vi "Chamber Engine.vi"(11 "Sequence Context In":refnum<k7>) -> (0 "error out":errorcluster)   [LabVIEW 2023, in "LTT_TeststandSteptypes.lvlib"]
uses:
  LTT_TeststandSteptypes.lvlib
  HardwareAbstractionLayer_LVOOP/Modbus TCP/Modbus TCP_class/Modbus TCP.lvclass
  Temperature Controller/Control/TC FGV Action.ctl
  75a4899f-3d6f-49ef-a0cc-877733f6873c.vi
  <vilib>/addons/TestStand/_TSUtility.llb/TestStand - Get Property Value (Boolean).vi
  GlobalVariable/GlobalVariableData.vi
  <vilib>/addons/TestStand/_TSUtility.llb/TestStand - Set Property Value (Number).vi
  HardwareAbstractionLayer_LVOOP/Teststand/Teststand.lvclass
  HardwareAbstractionLayer_LVOOP/Database/Database.lvclass
  HardwareAbstractionLayer_LVOOP/Modbus/Modbus_class/Modbus.lvclass
  HardwareAbstractionLayer_LVOOP/Database/SQL Public VI/Control/DB Options.ctl
panel:
  in  "stop":bool
  in  "error in (no error)":errorcluster
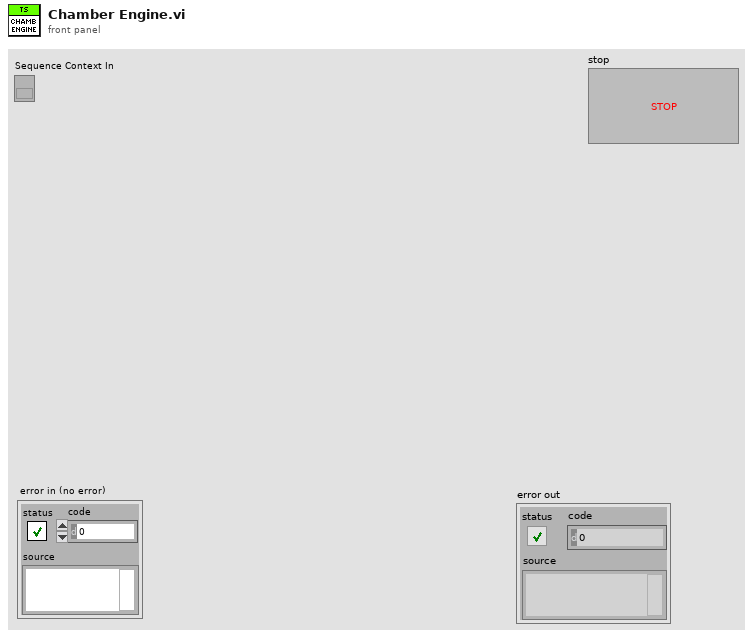
[diagram p1: front panel]
types:
  T1 = typedef "HardwareAbstractionLayer_LVOOP.lvlib/Database.lvclass/DB Options.ctl" = enum16{"Init", "Select Data", "Insert Data", "Update Data", "Delete Data", "Execute Query", "Create Schema", "Create Table", "List Tables", "List Columns", "Close"}
  T2 = typedef "LTT_TeststandSteptypes.lvlib/TC FGV Action.ctl" = enum16{"Set", "Get"}
  T3 = typedef "TestStand - Status Monitor.ctl" = cluster{"Sequence Context":refnum<k7>, "Execution":refnum<k7>, "Termination Monitor":refnum<k7>}
  T4 = typedef "HardwareAbstractionLayer_LVOOP.lvlib/Report.lvclass/Temperature LOG.ctl" = cluster{"TEST_MODE":string, "CYCLE_NUMBER":string, "TEMPERATURE":cluster{"LV_PPS_TEMPERATURE":dbl, "HV_PPS1_TEMPERATURE":dbl, "HV_PPS2_TEMPERATURE":dbl, "HV_PPS3_TEMPERATURE":dbl, "HV_PPS4_TEMPERATURE":dbl, "HV_PPS5_TEMPERATURE":dbl, "HV_PPS6_TEMPERATURE":dbl, "CHAMBER_TEMPERATURE":dbl, "LOAD_U1_TEMPERATURE":dbl, "LOAD_V1_TEMPERATURE":dbl, "LOAD_W1_TEMPERATURE":dbl, "LOAD_U2_TEMPERATURE":dbl, "LOAD_V2_TEMPERATURE":dbl, "LOAD_W2_TEMPERATURE":dbl, "LOAD_U3_TEMPERATURE":dbl, "LOAD_V3_TEMPERATURE":dbl, "LOAD_W3_TEMPERATURE":dbl}, "Temperature Inrange":cluster{"LVPPS_Trip?":bool, "HVPPS1_Trip?":bool, "HVPPS2_Trip?":bool, "HVPPS3_Trip?":bool, "HVPPS4_Trip?":bool, "HVPPS5_Trip?":bool, "HVPPS6_Trip?":bool, "Chamber_Trip?":bool}}
  T5 = cluster{"Chamber Present Temp":dbl, "Chamber Target Temp":dbl, "Chamber RTD Temp":dbl}
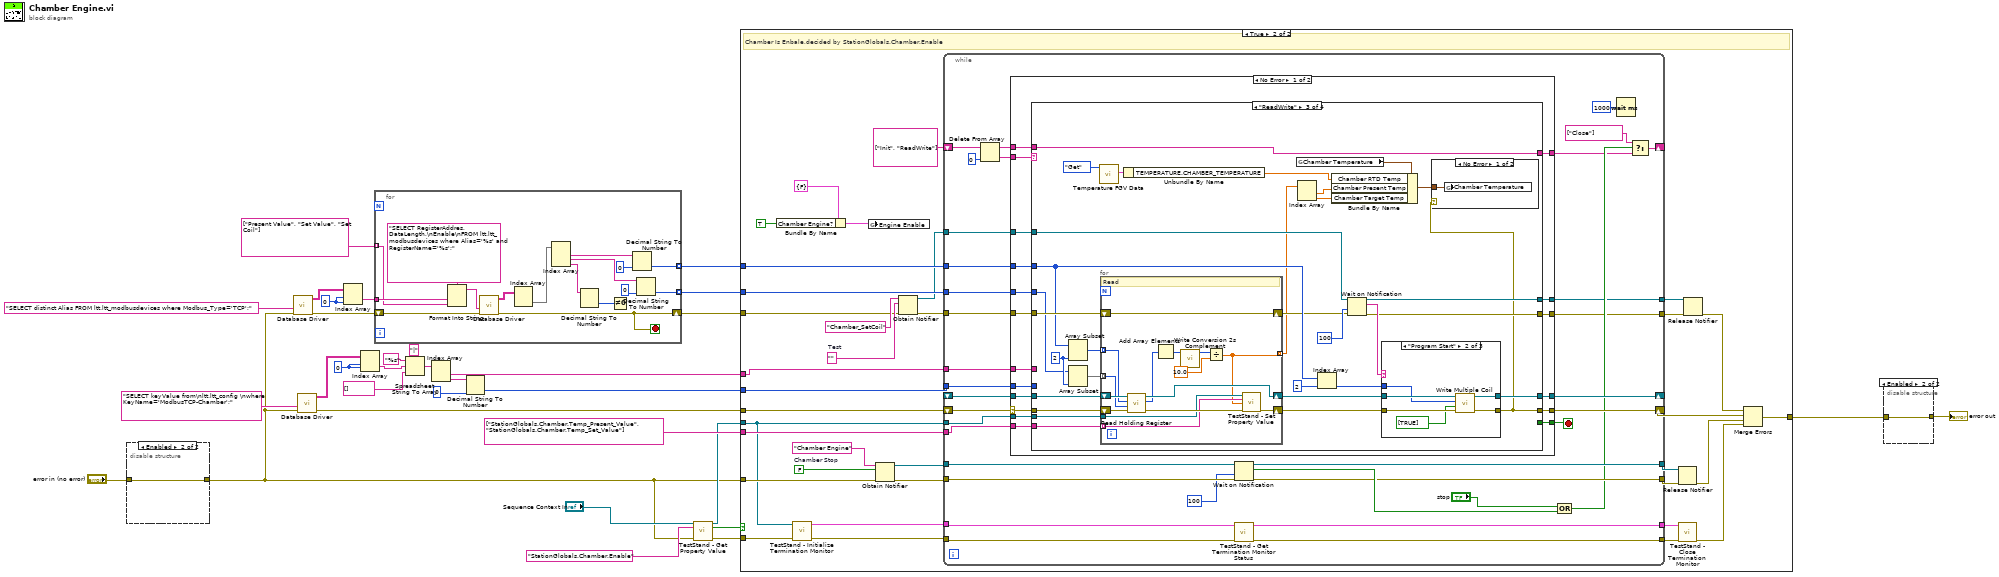
[diagram p0: block diagram]
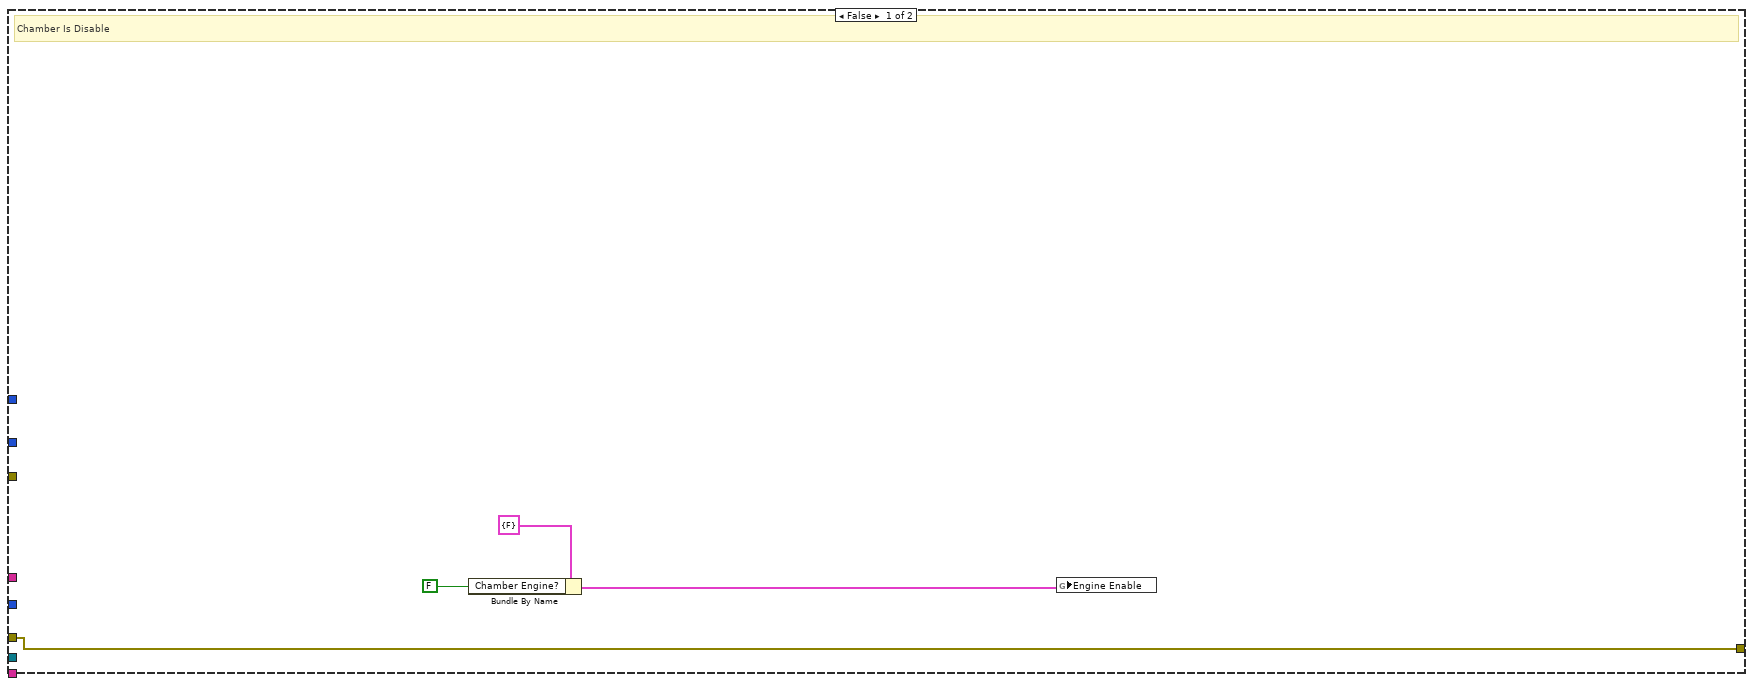
[diagram p2: hidden frame]
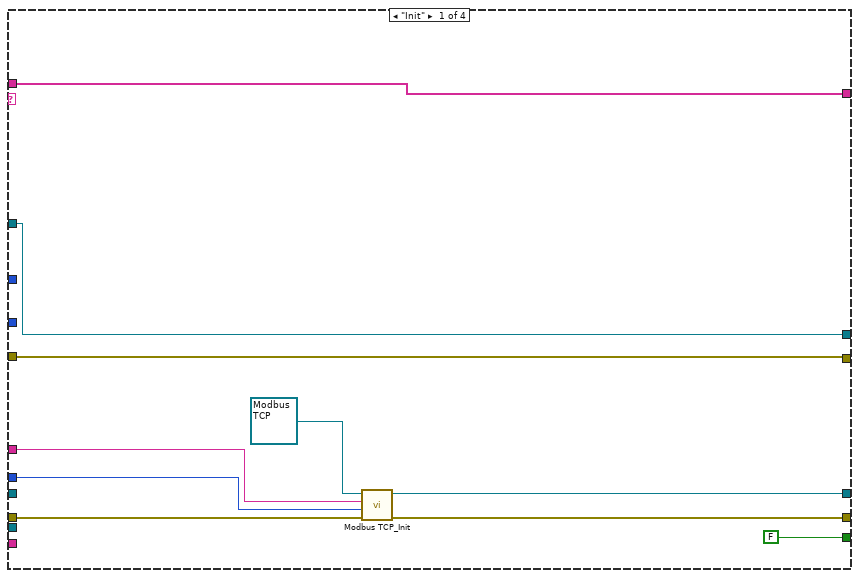
[diagram p3: hidden frame]
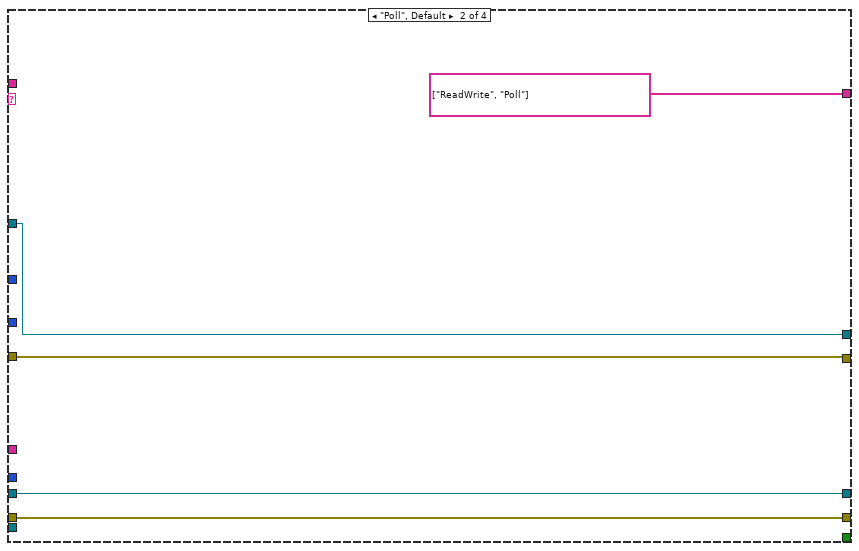
[diagram p4: hidden frame]
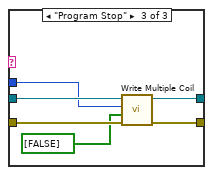
[diagram p7: hidden frame]
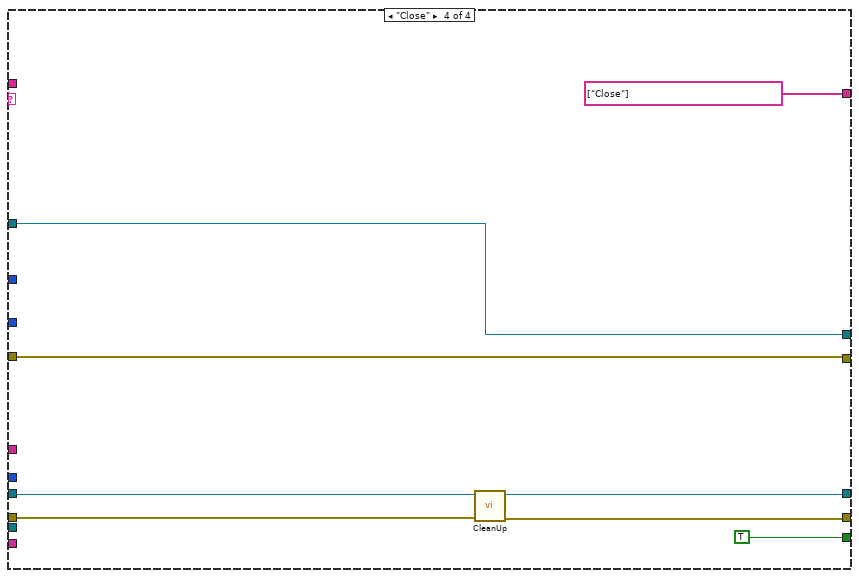
[diagram p8: hidden frame]
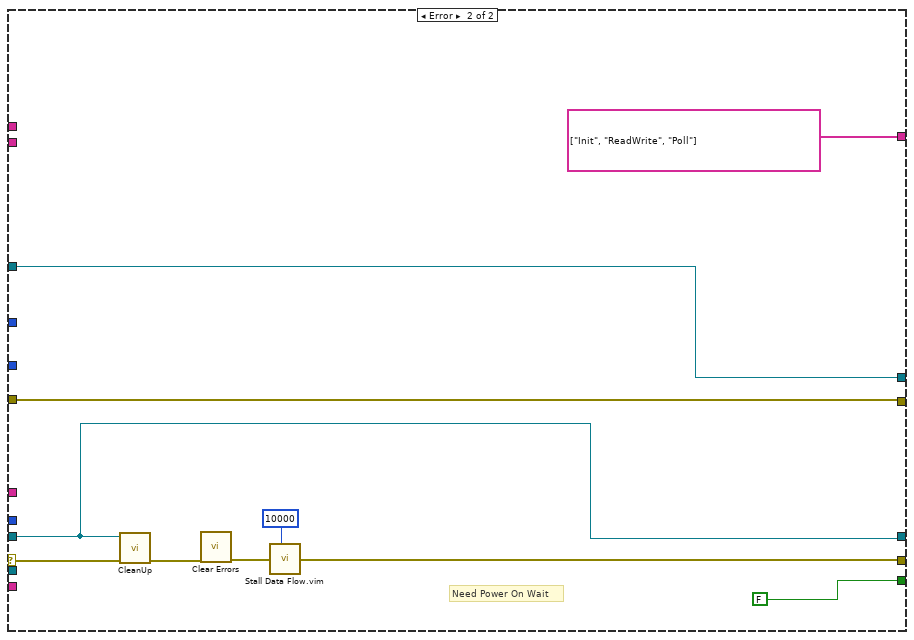
[diagram p9: hidden frame]
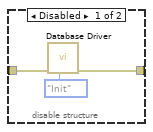
[diagram p10: hidden frame]
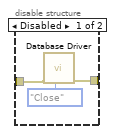
[diagram p11: hidden frame]
diagram:
  w17 = 0 ("disabled index (col)")
  w25 = 0 ("index (row)")
  n1 = disable-structure shown="Enabled" {
    disable-tunnel: "error in (no error)" -> [w34 w36]
    disable-tunnel: [w33 w36] -> w3
    frame Disabled {
      n2 = call "Database Driver.vi"("Options"=DB_Options."Init", "error in"=w34) -> ("error out"=w33:errorcluster)  [unwired: 6 in, 3 out]
    }
    frame Enabled {
    }
  }
  n3 = call "Database Driver.vi"("error in"=w3, "SQL query"="SELECT distinct Alias FROM ltt.ltt_modbusdevices where Modbus_Type='TCP';") -> ("error out"=w16:errorcluster, "data"=w18:string[][])  [unwired: 6 in, 2 out]
  n4 = call "Database Driver.vi"("error in"=w3, "SQL query"="SELECT keyValue from\nltt.ltt_config \nwhere KeyName='ModbusTCP-Chamber';") -> ("error out"=w20:errorcluster, "data"=w26:string[][])  [unwired: 6 in, 2 out]
  n5 = Index Array(array=w18, index (row)=w17, index (col)=w17) -> (element=w19:string)
  n6 = Index Array(array=w26, index (row)=w25, index (col)=w25) -> (element=w32:string)
  n7 = for {
    tunnel: w19 -> [w40]
    tunnel: [w46] -> w14 mode=indexing
    tunnel: [w45] -> w13 mode=indexing
    shift-right: [w44] -> w12
    shift-left: w16 -> [w43]
    tunnel: string[] ["Present Value", "Set Value", "Set Coil"] -> [w39] mode=indexing
    stop <- w44 stop-if-true
    n8 = Format Into String(format string="SELECT RegisterAddres, DataLength,\nEnable\nFROM ltt.ltt_modbusdevices where Alias='%s' and RegisterName='%s';", w40, w39) -> (resulting string=w52:string)  [unwired: 2 in, 1 out]
    n9 = call "Database Driver.vi"("error in"=w43, "SQL query"=w52) -> ("error out"=w44:errorcluster, "data"=w51:string[][])  [unwired: 6 in, 2 out]
    n10 = Index Array(array=w51) -> (element=w50:string[])  [unwired: 2 in]
    n11 = Index Array(array=w50) -> (element #1=w42:string, element #2=w41:string, element #3=w38:string)  [unwired: 3 in]
    n12 = Decimal String To Number(string=w38) -> (number=w37:i32)  [unwired: 2 in, 1 out]
    n13 = Not Equal To 0?(x=w37) -> ()  [unwired: 1 out]
    n14 = Decimal String To Number(string=w42, default (0L)=u16 0 ("starting address")) -> (number=w46:u16)  [unwired: 1 in, 1 out]
    n15 = Decimal String To Number(string=w41, default (0L)=u16 0 ("number of inputs")) -> (number=w45:u16)  [unwired: 1 in, 1 out]
  }
  n16 = Spreadsheet String To Array(delimiter (Tab)="|" ("format string"), format string="%s", spreadsheet string=w32, array type (2D Dbl)=string[] []) -> (array=w30:string[])
  n17 = Index Array(array=w30) -> (element #1=w21:string, element #2=w23:string)  [unwired: 2 in]
  n18 = Decimal String To Number(string=w23, default (0L)=u16 0 ("Port")) -> (number=w22:u16)  [unwired: 1 in, 1 out]
  n19 = call-poly <vilib>:"TestStand - Get Property Value.vi"("Sequence Context In"="Sequence Context In", "Lookup String"="StationGlobals.Chamber.Enable", "error in (no error)"=w3) -> ("Sequence Context Out"=w5:refnum<k7>, "Value"=w1:bool, "error out"=w2:errorcluster)  [unwired: 10 in]
  n20 = case shown="True" w1 {
    tunnel: w22 -> [_ w77]
    tunnel: w21 -> [_ w76]
    tunnel: w20 -> [w55 w75]
    tunnel: w14 -> [_ w74]
    tunnel: w13 -> [_ w73]
    tunnel: w12 -> [_ w70]
    tunnel: w3 -> [_ w64]
    tunnel: [w55 w63] -> w9
    tunnel: string[] ["StationGlobals.Chamber.Temp_Present_Value", "StationGlobals.Chamber.Temp_Set_Value"] -> [_ w59]
    tunnel: w5 -> [_ w56]
    tunnel: w2 -> [_ w57]
    frame False {
      w54 = cluster{"Chamber Engine?":bool} {"Chamber Engine?"=FALSE} ("Engine Enable")
      # "Chamber Is Disable"
      n21 = Bundle By Name(cluster=w54, "Chamber Engine?"=FALSE) -> ()  [unwired: 1 out]
      n22 = global write "GlobalVariableData.vi" "Engine Enable"(w54) -> ()
    }
    frame True {
      w71 = ""  # Test
      w89 = FALSE  # Chamber Stop
      # "Chamber Is Enbale,decided by StationGlobals.Chamber.Enable"
      n23 = Bundle By Name(cluster=cluster{"Chamber Engine?":bool} {"Chamber Engine?"=FALSE} ("Engine Enable"), "Chamber Engine?"=TRUE) -> (w60:cluster{"Chamber Engine?":bool})
      n24 = call <vilib>:"TestStand - Initialize Termination Monitor.vi"("error in (no error)"=w57, "Sequence Context In"=w56) -> ("error out"=w58:errorcluster, "Status Monitor Out"=w88:T3)  [unwired: 8 in]
      n25 = global write "GlobalVariableData.vi" "Engine Enable"(w60) -> ()
      n26 = Obtain Notifier(name (unnamed)="Chamber Engine", notification data type=w89, error in (no error)=w64) -> (notifier out=w86:refnum<notifier>, error out=w87:errorcluster)  [unwired: 1 in, 1 out]
      n27 = Obtain Notifier(name (unnamed)="Chamber_SetCoil", notification data type=w71, error in (no error)=w70) -> (notifier out=w68:refnum<notifier>, error out=w69:errorcluster)  [unwired: 1 in, 1 out]
      n28 = while {
        tunnel: w58 -> [w118]
        tunnel: w88 -> [w119]
        tunnel: w87 -> [w120]
        tunnel: w86 -> [w121]
        tunnel: [w114] -> w83
        tunnel: [w113] -> w84
        shift-right: [w123] -> _
        shift-left: _ -> [w125]
        shift-right: [w122] -> w85
        shift-left: w75 -> [w124]
        tunnel: [w112] -> w82
        tunnel: [w110] -> w81
        tunnel: w77 -> [w109]
        shift-right: [w100] -> _
        shift-left: string[] ["Init", "ReadWrite"] -> [w108]
        tunnel: w76 -> [w104]
        tunnel: w74 -> [w98]
        tunnel: w73 -> [w97]
        tunnel: w69 -> [w96]
        tunnel: w68 -> [w95]
        tunnel: [w94] -> w67
        tunnel: [w93] -> w66
        tunnel: w59 -> [w92]
        tunnel: w56 -> [w91]
        stop <- w102 stop-if-true
        n29 = Delete From Array(array=w108, index=0) -> (deleted portion=w107:string, array with subset deleted=w106:string[])  [unwired: 1 in]
        n30 = case shown="No Error" w124 {
          selector: w124 -> [w142 w237]
          tunnel: w125 -> [w143 w228]
          tunnel: [w141 w228] -> w123
          tunnel: [w140 w234] -> w122
          tunnel: w109 -> [w128 _]
          tunnel: w107 -> [w139 _]
          tunnel: w106 -> [w138 _]
          tunnel: [w137 string[] ["Init", "ReadWrite", "Poll"]] -> w101
          tunnel: w104 -> [w136 _]
          tunnel: [w135 FALSE] -> w102
          tunnel: w98 -> [w134 _]
          tunnel: w97 -> [w133 _]
          tunnel: w96 -> [w132 w229]
          tunnel: w95 -> [w131 w230]
          tunnel: [w130 w230] -> w93
          tunnel: [w129 w229] -> w94
          tunnel: w91 -> [w127 _]
          tunnel: w92 -> [w126 _]
          frame No Error {
            n31 = case shown="\"ReadWrite\"" w139 {
              tunnel: w143 -> [_ w157 w189 w227]
              tunnel: w142 -> [w151 w156 w188 w226]
              tunnel: [w150 w157 w185 w224] -> w141
              tunnel: [w149 w156 w161 w225] -> w140
              tunnel: w138 -> [w148 _ w184 _]
              tunnel: [w148 string[] ["ReadWrite", "Poll"] w184 string[] ["Close"]] -> w137
              tunnel: w136 -> [w153 _ _ _]
              tunnel: [FALSE _ _ TRUE] -> w135
              tunnel: w134 -> [_ _ w178 _]
              tunnel: w133 -> [_ _ w177 _]
              tunnel: w132 -> [w146 w155 w180 w221]
              tunnel: w131 -> [w145 w154 w179 w220]
              tunnel: [w145 w154 w172 w220] -> w130
              tunnel: [w146 w155 w171 w221] -> w129
              tunnel: w128 -> [w144 _ _ _]
              tunnel: w127 -> [_ _ w170 _]
              tunnel: w126 -> [_ _ w169 _]
              frame "Init" {
                n32 = call "Modbus TCP_Init.vi"("error in (no error)"=w151, "Port"=w144, "Slave Address"=w153, "object in"=refnum<class "Modbus TCP.lvclass"> refnum) -> ("error out"=w149:errorcluster, "object out"=w150:refnum<class "Modbus TCP.lvclass">)  [unwired: 6 in]
              }
              frame "Poll", Default {
              }
              frame "ReadWrite" {
                w183 = 2 ("length")
                n33 = Array Subset(array=w178, length=w183) -> (w182:u16[])  [unwired: 1 in]
                n34 = Array Subset(array=w177, length=w183) -> (w181:u16[])  [unwired: 1 in]
                n35 = call "Temperature FGV Data.vi"("Action"=TC_FGV_Action."Get") -> ("Temperature log Out"=w165:T4)  [unwired: 9 in, 1 out]
                n36 = for {
                  shift-right: [w217] -> w187
                  shift-left: w189 -> [w219]
                  shift-right: [w208] -> w186
                  shift-left: w188 -> [w218]
                  tunnel: w182 -> [w214] mode=indexing
                  tunnel: w181 -> [w213] mode=indexing
                  shift-right: [w212] -> w166
                  shift-left: w180 -> [w212]
                  tunnel: w170 -> [w207]
                  tunnel: w169 -> [w206] mode=indexing
                  tunnel: [w205] -> w164 mode=indexing
                  # "Read"
                  n37 = call-dynamic "Read Holding Register.vi"("error in (no error)"=w218, "number of inputs"=w213, "starting address"=w214, "Modbus TCP in"=w219) -> ("error out"=w209:errorcluster, "register values"=w215:u16[], "Modbus TCP out"=w217:refnum<class "Modbus TCP.lvclass">)  [unwired: 5 in]
                  n38 = Add Array Elements(numeric array=w215) -> (sum=w211:u16)
                  n39 = call "Write Conversion 2s Complement.vi"("Set Data Input"=w211) -> ("Coversion Data Output"=w210:i16)  [unwired: 10 in]
                  n40 = Divide(x=w210, y=10.0) -> (x/y=w205:dbl)
                  n41 = call-poly <vilib>:"TestStand - Set Property Value.vi"("Sequence Context In"=w207, "Lookup String"=w206, "New Value"=w205, "error in (no error)"=w209) -> ("error out"=w208:errorcluster)  [unwired: 10 in, 1 out]
                }
                n42 = Unbundle By Name(w165) -> ("TEMPERATURE.CHAMBER_TEMPERATURE"=w159:dbl)
                n43 = global read "GlobalVariableData.vi" "Chamber Temperature"() -> (w160:T5)
                n44 = Index Array(array=w164) -> (element #1=w163:dbl, element #2=w162:dbl)  [unwired: 2 in]
                n45 = Index Array(array=w178, index=2) -> (element=w175:u16)
                n46 = Bundle By Name(cluster=w160, "Chamber RTD Temp"=w159, "Chamber Present Temp"=w163, "Chamber Target Temp"=w162) -> (w168:T5)
                n47 = Wait on Notification(notifier=w179, timeout in ms (-1)=100, error in (no error)=w166) -> (notifier out=w172:refnum<notifier>, notification=w173:string, error out=w171:errorcluster)  [unwired: 1 in, 1 out]
                n48 = case shown="\"Program Start\"" w173 {
                  tunnel: w187 -> [w192 w198 w204]
                  tunnel: w186 -> [w191 w197 w203]
                  tunnel: [w192 w196 w202] -> w185
                  tunnel: [w191 w195 w201] -> w161
                  tunnel: w175 -> [_ w194 w200]
                  frame "", Default {
                  }
                  frame "Program Start" {
                    n49 = call-dynamic "Write Multiple Coil.vi"("error in (no error)"=w197, "coils to write"=bool[] [TRUE], "starting address"=w194, "Modbus TCP in"=w198) -> ("error out"=w195:errorcluster, "Modbus TCP out"=w196:refnum<class "Modbus TCP.lvclass">)  [unwired: 6 in]
                  }
                  frame "Program Stop" {
                    n50 = call-dynamic "Write Multiple Coil.vi"("error in (no error)"=w203, "coils to write"=bool[] [FALSE], "starting address"=w200, "Modbus TCP in"=w204) -> ("error out"=w201:errorcluster, "Modbus TCP out"=w202:refnum<class "Modbus TCP.lvclass">)  [unwired: 6 in]
                  }
                }
                n51 = case shown="No Error" w161 {
                  tunnel: w168 -> [w190 _]
                  frame No Error {
                    n52 = global write "GlobalVariableData.vi" "Chamber Temperature"(w190) -> ()
                  }
                  frame Error {
                  }
                }
              }
              frame "Close" {
                n53 = call-dynamic "CleanUp.vi"("error in (no error)"=w226, "object in"=w227) -> ("error out"=w225:errorcluster, "object out"=w224:refnum<class "Modbus TCP.lvclass">)  [unwired: 8 in]
              }
            }
          }
          frame Error {
            # "Need Power On Wait"
            n54 = call-dynamic "CleanUp.vi"("error in (no error)"=w237, "object in"=w228) -> ("error out"=w236:errorcluster)  [unwired: 8 in, 1 out]
            n55 = call <vilib>:"Clear Errors.vi"("error in (no error)"=w236) -> ("error out"=w235:errorcluster)  [unwired: 5 in, 1 out]
            n56 = call "Stall Data Flow.vim"("value in"=w235, "milliseconds to wait"=u32 10000) -> ("value out"=w234:errorcluster)  [unwired: 1 out]
          }
        }
        n57 = Wait on Notification(notifier=w121, timeout in ms (-1)=100, error in (no error)=w120) -> (notifier out=w112:refnum<notifier>, notification=w117:bool, error out=w110:errorcluster)  [unwired: 1 in, 1 out]
        n58 = call <vilib>:"TestStand - Get Termination Monitor Status.vi"("error in (no error)"=w118, "Status Monitor In"=w119) -> ("error out"=w114:errorcluster, "Status Monitor Out"=w113:T3)  [unwired: 7 in, 1 out]
        n59 = Compound Arithmetic op=OR("stop", w117) -> (w103:bool)
        n60 = Wait (ms)(milliseconds to wait=u32 1000) -> ()  [unwired: 1 out]
        n61 = Select(t=string[] ["Close"], s=w103, f=w101) -> (s? t:f=w100:string[])
      }
      n62 = Release Notifier(notifier=w82, error in (no error)=w81) -> (error out=w80:errorcluster)  [unwired: 1 in, 2 out]
      n63 = call <vilib>:"TestStand - Close Termination Monitor.vi"("error in (no error)"=w83, "Status Monitor In"=w84) -> ("error out"=w79:errorcluster)  [unwired: 9 in]
      n64 = Release Notifier(notifier=w66, error in (no error)=w67) -> (error out=w65:errorcluster)  [unwired: 1 in, 2 out]
      n65 = Merge Errors(w65, w85, w80, w79) -> (w63:errorcluster)
    }
  }
  n66 = disable-structure shown="Enabled" {
    disable-tunnel: w9 -> [w239 w241]
    disable-tunnel: [w238 w241] -> w8
    frame Disabled {
      n67 = call "Database Driver.vi"("Options"=DB_Options."Close", "error in"=w239) -> ("error out"=w238:errorcluster)  [unwired: 6 in, 3 out]
    }
    frame Enabled {
    }
  }
  "error out" <- w8
